vi "unit.vi"(8 "Error In":errorcluster, 9 "Signal Amp":dbl format="%#_7f", 11 "Unit":string) -> (0 "Error Out":errorcluster)   [LabVIEW 2021, in "Signal.lvlib"]
doc: "This subVI is used to check the unit value range and to enter the values to the signal_values_FGV."
uses:
  Signal.lvlib
  Tipski Definicii/rel_error.ctl
  Tipski Definicii/Unit.ctl
  Tipski Definicii/Signal Values.ctl
panel:
  # "Input"
  # "Output"
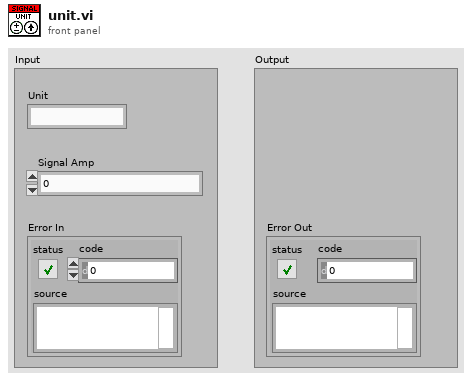
[diagram p1: front panel]
types:
  T1 = typedef "Unit.ctl" = enum16{"Init", "Add", "Read"}
  T2 = typedef "rel_error.ctl" = enum16{"Init", "Add String", "Error", "Get Error and Strings", "Reset"}
  T3 = typedef "Signal Values.ctl" = enum16{"Init", "Add V/A string", "Add Hz string", "Get Strings and Values", "Reset", "Add Offset", "Add Waveform", "Add Phase"}
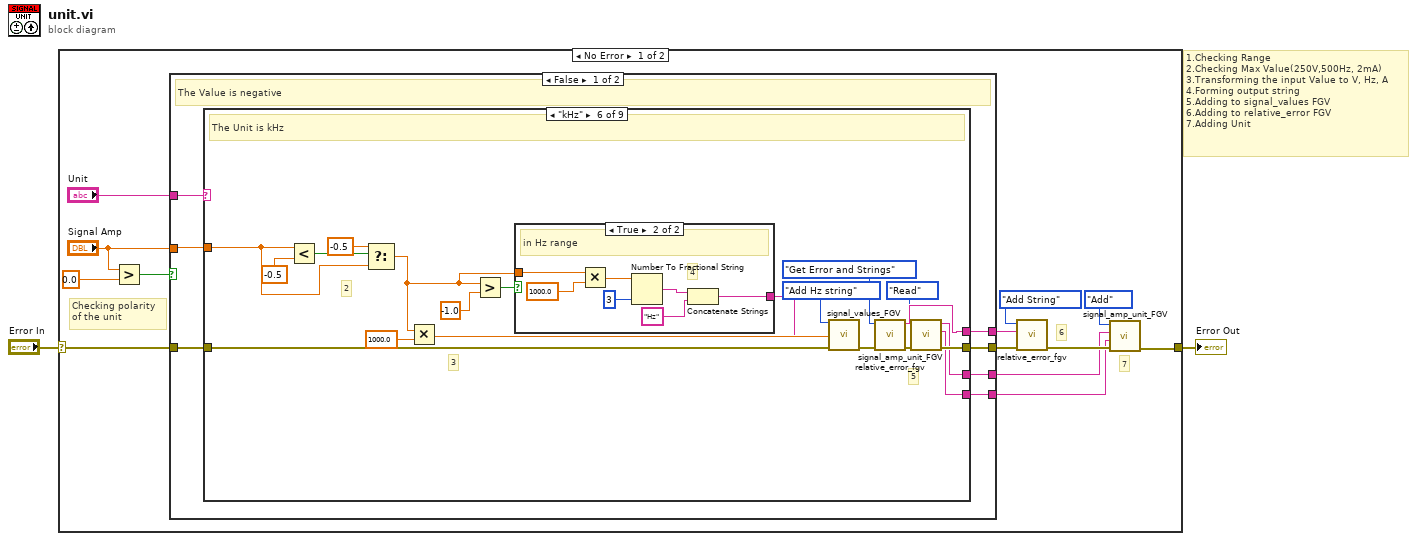
[diagram p0: block diagram]
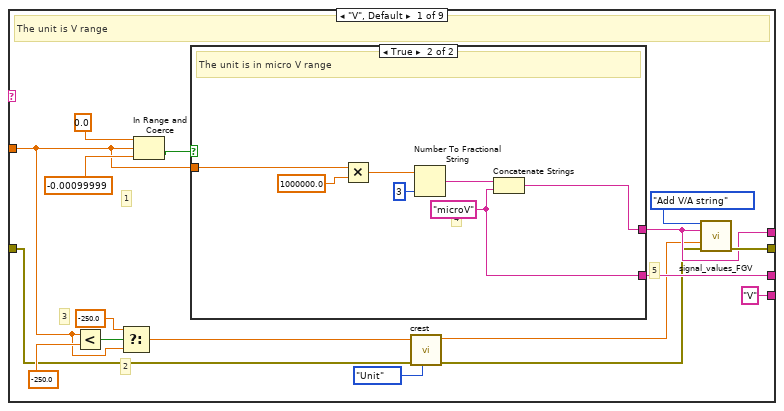
[diagram p2: hidden frame]
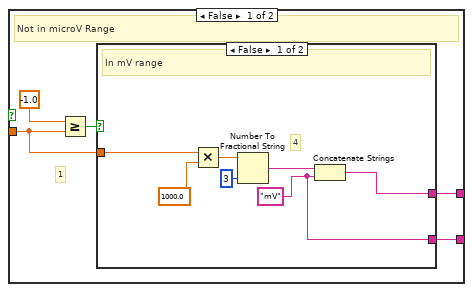
[diagram p3: hidden frame]
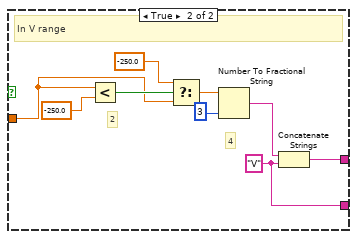
[diagram p4: hidden frame]
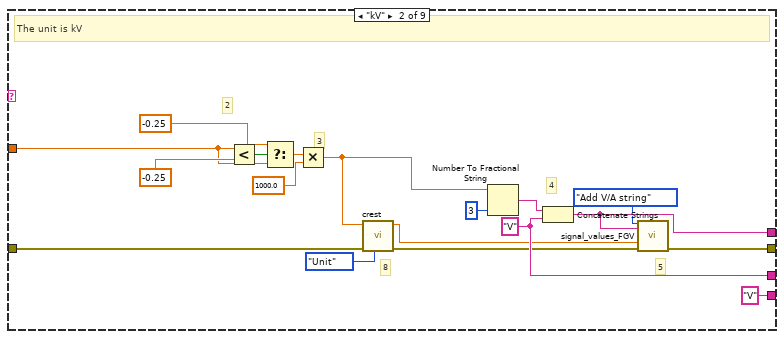
[diagram p5: hidden frame]
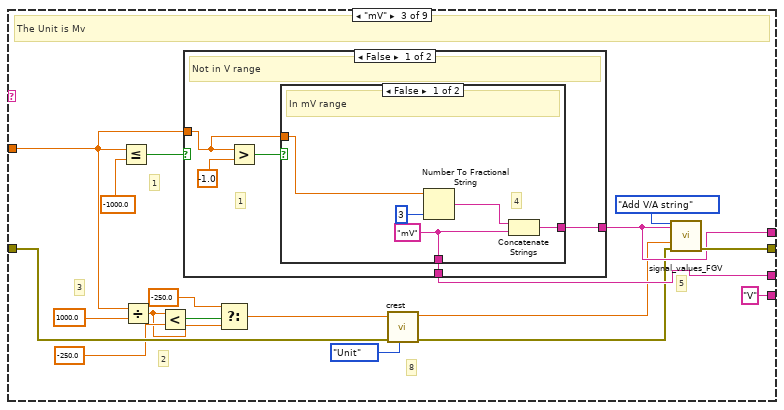
[diagram p6: hidden frame]
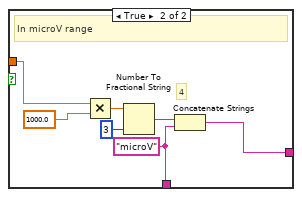
[diagram p7: hidden frame]
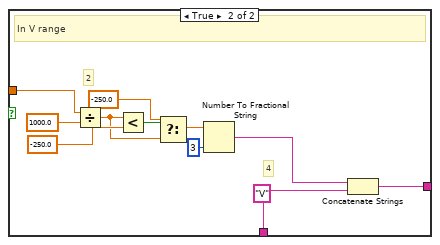
[diagram p8: hidden frame]
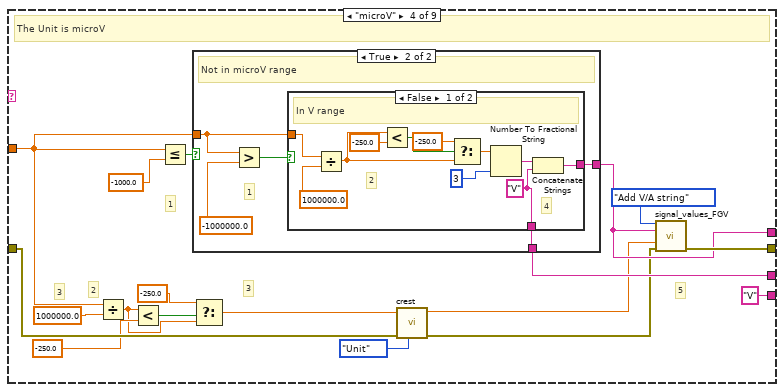
[diagram p9: hidden frame]
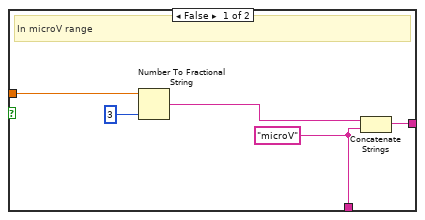
[diagram p10: hidden frame]
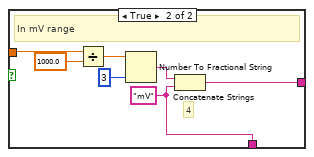
[diagram p11: hidden frame]
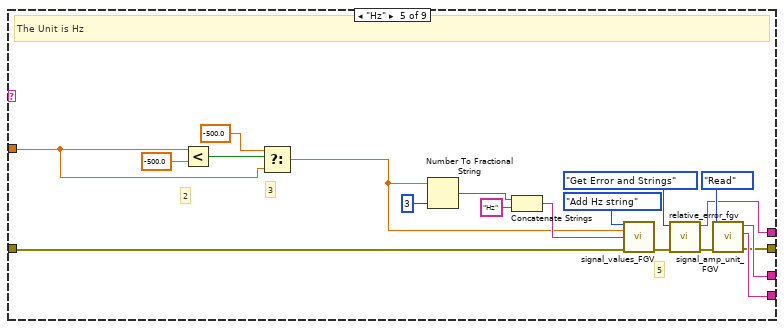
[diagram p12: hidden frame]
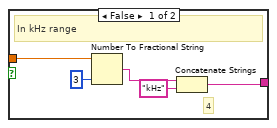
[diagram p13: hidden frame]
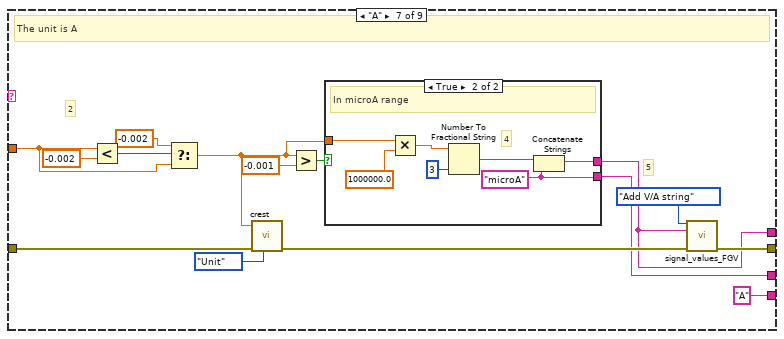
[diagram p14: hidden frame]
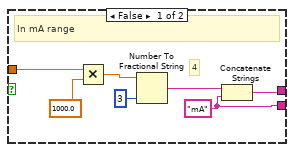
[diagram p15: hidden frame]
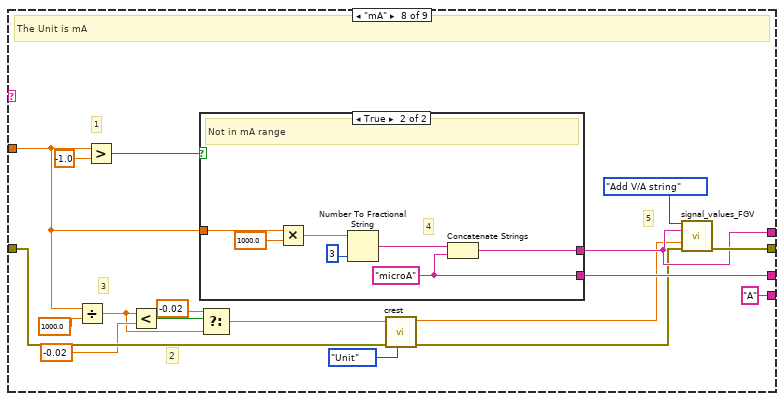
[diagram p16: hidden frame]
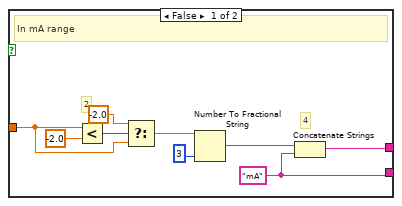
[diagram p17: hidden frame]
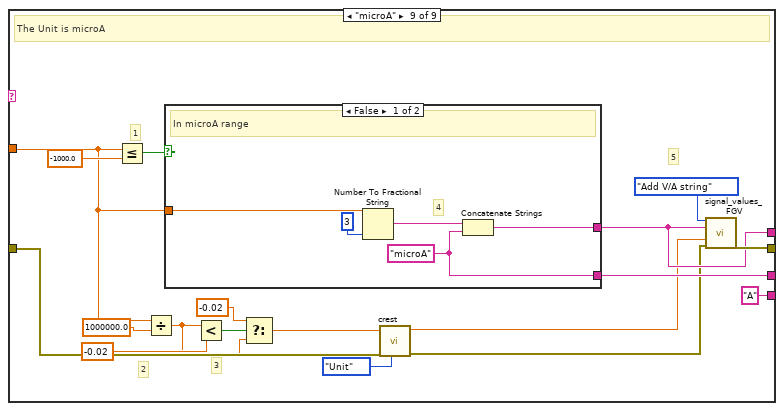
[diagram p18: hidden frame]
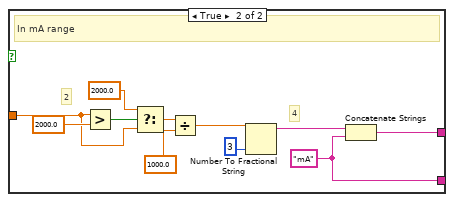
[diagram p19: hidden frame]
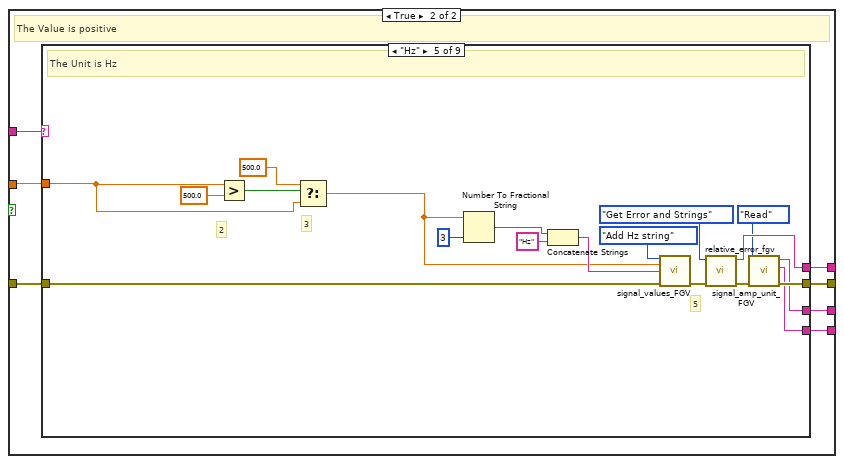
[diagram p20: hidden frame]
diagram:
  # "1.Checking Range\n2.Checking Max Value(250V,500Hz, 2mA)\n3.Transforming the input Value to V, Hz, A\n4.Forming output string\n5.Adding to signal_values FGV\n6.Adding to relative_error FGV\n7.Adding Unit"
  n1 = case shown="No Error" "Error In" {
    selector: "Error In" -> [w14 w636]
    tunnel: [w4 w636] -> w1
    frame No Error {
      # "7"
      # "6"
      # "Checking polarity\nof the unit"
      n2 = Greater?(x="Signal Amp", y=0.0) -> (0:w12:bool)
      n3 = case shown="False" w12 {
        tunnel: "Unit" -> [w20 w332]
        tunnel: w14 -> [w22 w330]
        tunnel: "Signal Amp" -> [w21 w331]
        tunnel: [w18 w329] -> w10
        tunnel: [w17 w328] -> w9
        tunnel: [w19 w327] -> w5
        tunnel: [w16 w326] -> w3
        frame False {
          # "The Value is negative"
          n4 = case shown="\"kHz\"" w20 {
            tunnel: [w36 w85 w99 w146 w179 w201 w231 w272 w306] -> w18
            tunnel: w21 -> [w29 w81 w94 w140 w183 w206 w234 w269 w302]
            tunnel: w22 -> [w28 w73 w103 w149 w182 w207 w235 w275 w309]
            tunnel: [w35 w76 w93 w139 w178 w199 w230 w268 w301] -> w17
            tunnel: [w34 w75 w92 w138 w180 w200 w232 w267 w304] -> w19
            tunnel: ["V" ("Base") "V" ("Base") "V" ("Base") "V" ("Base") w181 w197 "A" ("Base") "A" ("Base") "A" ("Base")] -> w16
            frame "V", Default {
              # "3"
              # "2"
              # "5"
              # "1"
              # "The unit is V range"
              n5 = Less?(x=w29, y=-250.0) -> (x < y?=w31:bool)
              n6 = Select(t=-250.0, s=w31, f=w29) -> (s? t:f=w27:dbl)
              n7 = In Range and Coerce(upper limit=0.0, x=w29, lower limit=-0.00099999) -> (In Range?=w39:bool)  [unwired: 1 out]
              n8 = case shown="True" w39 {
                tunnel: w29 -> [w42 w67]
                tunnel: [w41 w63] -> w35
                tunnel: [w40 w62] -> w34
                frame False {
                  # "1"
                  # "Not in microV Range"
                  n9 = Greater Or Equal?(x=-1.0, y=w42) -> (x >= y?=w43:bool)
                  n10 = case shown="False" w43 {
                    tunnel: w42 -> [w51 w56]
                    tunnel: [w47 w54] -> w41
                    tunnel: [w46 w53] -> w40
                    frame False {
                      w46 = "mV" ("string")
                      # "4"
                      # "In mV range"
                      n11 = Multiply(x=w51, y=1000.0) -> (x*y=w45:dbl)
                      n12 = Number To Fractional String(number=w45, precision (6)=i16 3) -> (F-format string=w48:string)  [unwired: 2 in]
                      n13 = Concatenate Strings(w48, w46) -> (w47:string)
                    }
                    frame True {
                      w53 = "V" ("string")
                      # "2"
                      # "4"
                      # "In V range"
                      n14 = Less?(x=w56, y=-250.0) -> (x < y?=w59:bool)
                      n15 = Select(t=-250.0, s=w59, f=w56) -> (s? t:f=w52:dbl)
                      n16 = Number To Fractional String(number=w52, precision (6)=i16 3) -> (F-format string=w55:string)  [unwired: 2 in]
                      n17 = Concatenate Strings(w55, w53) -> (w54:string)
                    }
                  }
                }
                frame True {
                  w62 = "microV" ("string")
                  # "4"
                  # "The unit is in micro V range"
                  n18 = Multiply(x=w67, y=1000000.0) -> (x*y=w61:dbl)
                  n19 = Number To Fractional String(number=w61, precision (6)=i16 3) -> (F-format string=w64:string)  [unwired: 2 in]
                  n20 = Concatenate Strings(w64, w62) -> (w63:string)
                }
              }
              n21 = call "crest.vi"("Set / Unit?"=enum16{"Unit", "SetUp"}."Unit", "Error In"=w28, "RMS"=w27) -> ("Error Out"=w25:errorcluster, "Max"=w26:dbl)  [unwired: 7 in]
              n22 = call "signal_values_FGV.vi"("Action"=Signal_Values."Add V/A string", "Amp String"=w35, "Amp Value"=w26, "Error In"=w25) -> ("Error Out"=w36:errorcluster)  [unwired: 10 in, 1 out]
            }
            frame "kV" {
              w75 = "V" ("string")
              # "8"
              # "2"
              # "5"
              # "4"
              # "3"
              # "The unit is kV"
              n23 = Less?(x=w81, y=-0.25) -> (x < y?=w83:bool)
              n24 = Select(t=-0.25, s=w83, f=w81) -> (s? t:f=w80:dbl)
              n25 = Multiply(x=w80, y=1000.0) -> (x*y=w72:dbl)
              n26 = call "crest.vi"("Set / Unit?"=enum16{"Unit", "SetUp"}."Unit", "Error In"=w73, "RMS"=w72) -> ("Error Out"=w71:errorcluster, "Max"=w70:dbl)  [unwired: 7 in]
              n27 = Number To Fractional String(number=w72, precision (6)=i16 3) -> (F-format string=w77:string)  [unwired: 2 in]
              n28 = Concatenate Strings(w77, w75) -> (w76:string)
              n29 = call "signal_values_FGV.vi"("Action"=Signal_Values."Add V/A string", "Amp String"=w76, "Amp Value"=w70, "Error In"=w71) -> ("Error Out"=w85:errorcluster)  [unwired: 10 in, 1 out]
            }
            frame "mV" {
              # "8"
              # "5"
              # "1"
              # "3"
              # "2"
              # "The Unit is Mv"
              n30 = Less Or Equal?(x=w94, y=-1000.0) -> (x <= y?=w101:bool)
              n31 = Divide(x=w94, y=1000.0) -> (x/y=w95:dbl)
              n32 = Less?(x=w95, y=-250.0) -> (x < y?=w97:bool)
              n33 = case shown="False" w101 {
                tunnel: w94 -> [w106 w124]
                tunnel: [w105 w122] -> w93
                tunnel: [w104 w121] -> w92
                frame False {
                  # "1"
                  # "Not in V range"
                  n34 = Greater?(x=w106, y=-1.0) -> (0:w107:bool)
                  n35 = case shown="False" w107 {
                    tunnel: w106 -> [w110 w120]
                    tunnel: [w112 w116] -> w105
                    tunnel: [w109 w114] -> w104
                    frame False {
                      w109 = "mV" ("string")
                      # "4"
                      # "In mV range"
                      n36 = Number To Fractional String(number=w110, precision (6)=i16 3) -> (F-format string=w111:string)  [unwired: 2 in]
                      n37 = Concatenate Strings(w111, w109) -> (w112:string)
                    }
                    frame True {
                      w114 = "microV" ("string")
                      # "4"
                      # "In microV range"
                      n38 = Multiply(x=w120, y=1000.0) -> (x*y=w115:dbl)
                      n39 = Number To Fractional String(number=w115, precision (6)=i16 3) -> (F-format string=w117:string)  [unwired: 2 in]
                      n40 = Concatenate Strings(w117, w114) -> (w116:string)
                    }
                  }
                }
                frame True {
                  w121 = "V" ("string")
                  # "2"
                  # "4"
                  # "In V range"
                  n41 = Divide(x=w124, y=1000.0) -> (x/y=w125:dbl)
                  n42 = Less?(x=w125, y=-250.0) -> (x < y?=w127:bool)
                  n43 = Select(t=-250.0, s=w127, f=w125) -> (s? t:f=w123:dbl)
                  n44 = Number To Fractional String(number=w123, precision (6)=i16 3) -> (F-format string=w129:string)  [unwired: 2 in]
                  n45 = Concatenate Strings(w129, w121) -> (w122:string)
                }
              }
              n46 = Select(t=-250.0, s=w97, f=w95) -> (s? t:f=w90:dbl)
              n47 = call "crest.vi"("Set / Unit?"=enum16{"Unit", "SetUp"}."Unit", "Error In"=w103, "RMS"=w90) -> ("Error Out"=w88:errorcluster, "Max"=w89:dbl)  [unwired: 7 in]
              n48 = call "signal_values_FGV.vi"("Action"=Signal_Values."Add V/A string", "Amp String"=w93, "Amp Value"=w89, "Error In"=w88) -> ("Error Out"=w99:errorcluster)  [unwired: 10 in, 1 out]
            }
            frame "microV" {
              # "3"
              # "5"
              # "1"
              # "3"
              # "2"
              # "The Unit is microV"
              n49 = Divide(x=w140, y=1000000.0) -> (x/y=w141:dbl)
              n50 = Less?(x=w141, y=-250.0) -> (x < y?=w143:bool)
              n51 = Less Or Equal?(x=w140, y=-1000.0) -> (x <= y?=w147:bool)
              n52 = case shown="True" w147 {
                tunnel: [w152 w157] -> w139
                tunnel: w140 -> [w151 w156]
                tunnel: [w150 w155] -> w138
                frame False {
                  w150 = "microV" ("string")
                  # "In microV range"
                  n53 = Number To Fractional String(number=w151, precision (6)=i16 3) -> (F-format string=w154:string)  [unwired: 2 in]
                  n54 = Concatenate Strings(w154, w150) -> (w152:string)
                }
                frame True {
                  # "1"
                  # "Not in microV range"
                  n55 = Greater?(x=w156, y=-1000000.0) -> (0:w158:bool)
                  n56 = case shown="False" w158 {
                    tunnel: [w164 w176] -> w157
                    tunnel: w156 -> [w162 w173]
                    tunnel: [w160 w171] -> w155
                    frame False {
                      w160 = "V"
                      # "2"
                      # "4"
                      # "In V range"
                      n57 = Divide(x=w162, y=1000000.0) -> (x/y=w166:dbl)
                      n58 = Less?(x=w166, y=-250.0) -> (x < y?=w168:bool)
                      n59 = Select(t=-250.0, s=w168, f=w166) -> (s? t:f=w161:dbl)
                      n60 = Number To Fractional String(number=w161, precision (6)=i16 3) -> (F-format string=w165:string)  [unwired: 2 in]
                      n61 = Concatenate Strings(w165, w160) -> (w164:string)
                    }
                    frame True {
                      w171 = "mV"
                      # "4"
                      # "In mV range"
                      n62 = Divide(x=w173, y=1000.0) -> (x/y=w172:dbl)
                      n63 = Number To Fractional String(number=w172, precision (6)=i16 3) -> (F-format string=w175:string)  [unwired: 2 in]
                      n64 = Concatenate Strings(w175, w171) -> (w176:string)
                    }
                  }
                }
              }
              n65 = Select(t=-250.0, s=w143, f=w141) -> (s? t:f=w136:dbl)
              n66 = call "crest.vi"("Set / Unit?"=enum16{"Unit", "SetUp"}."Unit", "Error In"=w149, "RMS"=w136) -> ("Error Out"=w134:errorcluster, "Max"=w135:dbl)  [unwired: 7 in]
              n67 = call "signal_values_FGV.vi"("Action"=Signal_Values."Add V/A string", "Amp String"=w139, "Amp Value"=w135, "Error In"=w134) -> ("Error Out"=w146:errorcluster)  [unwired: 10 in, 1 out]
            }
            frame "Hz" {
              # "5"
              # "3"
              # "2"
              # "The Unit is Hz"
              n68 = Less?(x=w183, y=-500.0) -> (x < y?=w195:bool)
              n69 = Select(t=-500.0 ("y"), s=w195, f=w183) -> (s? t:f=w184:dbl)
              n70 = Number To Fractional String(number=w184, precision (6)=i16 3) -> (F-format string=w186:string)  [unwired: 2 in]
              n71 = Concatenate Strings(w186, "Hz" ("string")) -> (w185:string)
              n72 = call "signal_values_FGV.vi"("Action"=Signal_Values."Add Hz string", "Hz Value"=w184, "Hz String"=w185, "Error In"=w182) -> ("Error Out"=w193:errorcluster)  [unwired: 10 in, 1 out]
              n73 = call "relative_error_fgv.vi"("Error In"=w193, "Action"=rel_error."Get Error and Strings") -> ("Error Out"=w190:errorcluster, "Starting String"=w178:string)  [unwired: 5 in, 3 out]
              n74 = call "signal_amp_unit_FGV.vi"("Error In"=w190, "Action"=Unit."Read") -> ("Error Out"=w179:errorcluster, "Base"=w181:string, "Unit (Not F)"=w180:string)  [unwired: 7 in]
            }
            frame "kHz" {
              # "5"
              # "3"
              # "2"
              # "The Unit is kHz"
              n75 = Less?(x=w206, y=-0.5) -> (x < y?=w215:bool)
              n76 = Select(t=-0.5, s=w215, f=w206) -> (s? t:f=w209:dbl)
              n77 = Multiply(x=w209, y=1000.0) -> (x*y=w212:dbl)
              n78 = Greater?(x=w209, y=-1.0) -> (0:w210:bool)
              n79 = case shown="True" w210 {
                tunnel: w209 -> [w221 w227]
                tunnel: [w217 w223] -> w208
                frame False {
                  # "4"
                  # "In kHz range"
                  n80 = Number To Fractional String(number=w221, precision (6)=i16 3) -> (F-format string=w219:string)  [unwired: 2 in]
                  n81 = Concatenate Strings(w219, "kHz" ("string")) -> (w217:string)
                }
                frame True {
                  # "4"
                  # "in Hz range"
                  n82 = Multiply(x=w227, y=1000.0) -> (x*y=w225:dbl)
                  n83 = Number To Fractional String(number=w225, precision (6)=i16 3) -> (F-format string=w228:string)  [unwired: 2 in]
                  n84 = Concatenate Strings(w228, "Hz" ("string")) -> (w223:string)
                }
              }
              n85 = call "signal_values_FGV.vi"("Action"=Signal_Values."Add Hz string", "Hz Value"=w212, "Hz String"=w208, "Error In"=w207) -> ("Error Out"=w205:errorcluster)  [unwired: 10 in, 1 out]
              n86 = call "relative_error_fgv.vi"("Error In"=w205, "Action"=rel_error."Get Error and Strings") -> ("Error Out"=w202:errorcluster, "Starting String"=w199:string)  [unwired: 5 in, 3 out]
              n87 = call "signal_amp_unit_FGV.vi"("Error In"=w202, "Action"=Unit."Read") -> ("Error Out"=w201:errorcluster, "Base"=w197:string, "Unit (Not F)"=w200:string)  [unwired: 7 in]
            }
            frame "A" {
              # "5"
              # "2"
              # "The unit is A"
              n88 = Less?(x=w234, y=-0.002) -> (x < y?=w242:bool)
              n89 = Select(t=-0.002, s=w242, f=w234) -> (s? t:f=w236:dbl)
              n90 = call "crest.vi"("Set / Unit?"=enum16{"Unit", "SetUp"}."Unit", "Error In"=w235, "RMS"=w236) -> ("Error Out"=w239:errorcluster)  [unwired: 7 in, 1 out]
              n91 = Greater?(x=w236, y=-0.001) -> (0:w237:bool)
              n92 = case shown="True" w237 {
                tunnel: [w245 w255] -> w232
                tunnel: [w244 w254] -> w230
                tunnel: w236 -> [w246 w253]
                frame False {
                  w245 = "mA" ("string")
                  # "4"
                  # "In mA range"
                  n93 = Multiply(x=w246, y=1000.0) -> (x*y=w248:dbl)
                  n94 = Number To Fractional String(number=w248, precision (6)=i16 3) -> (F-format string=w249:string)  [unwired: 2 in]
                  n95 = Concatenate Strings(w249, w245) -> (w244:string)
                }
                frame True {
                  w255 = "microA" ("string")
                  # "4"
                  # "In microA range"
                  n96 = Multiply(x=w253, y=1000000.0) -> (x*y=w252:dbl)
                  n97 = Number To Fractional String(number=w252, precision (6)=i16 3) -> (F-format string=w256:string)  [unwired: 2 in]
                  n98 = Concatenate Strings(w256, w255) -> (w254:string)
                }
              }
              n99 = call "signal_values_FGV.vi"("Action"=Signal_Values."Add V/A string", "Amp String"=w230, "Error In"=w239) -> ("Error Out"=w231:errorcluster)  [unwired: 11 in, 1 out]
            }
            frame "mA" {
              # "3"
              # "2"
              # "5"
              # "1"
              # "The Unit is mA"
              n100 = Divide(x=w269, y=1000.0) -> (x/y=w263:dbl)
              n101 = Greater?(x=w269, y=-1.0) -> (0:w273:bool)
              n102 = Less?(x=w263, y=-0.02) -> (x < y?=w265:bool)
              n103 = case shown="True" w273 {
                tunnel: w269 -> [w282 w291]
                tunnel: [w277 w287] -> w268
                tunnel: [w276 w286] -> w267
                frame False {
                  w276 = "mA" ("string")
                  # "4"
                  # "2"
                  # "In mA range"
                  n104 = Less?(x=w282, y=-2.0) -> (x < y?=w283:bool)
                  n105 = Select(t=-2.0, s=w283, f=w282) -> (s? t:f=w278:dbl)
                  n106 = Number To Fractional String(number=w278, precision (6)=i16 3) -> (F-format string=w279:string)  [unwired: 2 in]
                  n107 = Concatenate Strings(w279, w276) -> (w277:string)
                }
                frame True {
                  w286 = "microA" ("string")
                  # "4"
                  # "Not in mA range"
                  n108 = Multiply(x=w291, y=1000.0) -> (x*y=w288:dbl)
                  n109 = Number To Fractional String(number=w288, precision (6)=i16 3) -> (F-format string=w285:string)  [unwired: 2 in]
                  n110 = Concatenate Strings(w285, w286) -> (w287:string)
                }
              }
              n111 = Select(t=-0.02, s=w265, f=w263) -> (s? t:f=w261:dbl)
              n112 = call "crest.vi"("Set / Unit?"=enum16{"Unit", "SetUp"}."Unit", "Error In"=w275, "RMS"=w261) -> ("Error Out"=w262:errorcluster, "Max"=w260:dbl)  [unwired: 7 in]
              n113 = call "signal_values_FGV.vi"("Action"=Signal_Values."Add V/A string", "Amp String"=w268, "Amp Value"=w260, "Error In"=w262) -> ("Error Out"=w272:errorcluster)  [unwired: 10 in, 1 out]
            }
            frame "microA" {
              # "2"
              # "5"
              # "3"
              # "1"
              # "The Unit is microA"
              n114 = Less Or Equal?(x=w302, y=-1000.0) -> (x <= y?=w307:bool)
              n115 = Divide(x=w302, y=1000000.0) -> (x/y=w297:dbl)
              n116 = case shown="False" w307 {
                tunnel: w302 -> [w310 w322]
                tunnel: [w312 w316] -> w301
                tunnel: [w311 w315] -> w304
                frame False {
                  w311 = "microA" ("string")
                  # "4"
                  # "In microA range"
                  n117 = Number To Fractional String(number=w310, precision (6)=i16 3) -> (F-format string=w313:string)  [unwired: 2 in]
                  n118 = Concatenate Strings(w313, w311) -> (w312:string)
                }
                frame True {
                  w315 = "mA" ("string")
                  # "2"
                  # "4"
                  # "In mA range"
                  n119 = Greater?(x=w322, y=2000.0) -> (0:w324:bool)
                  n120 = Select(t=2000.0, s=w324, f=w322) -> (s? t:f=w321:dbl)
                  n121 = Divide(x=w321, y=1000.0) -> (x/y=w317:dbl)
                  n122 = Number To Fractional String(number=w317, precision (6)=i16 3) -> (F-format string=w318:string)  [unwired: 2 in]
                  n123 = Concatenate Strings(w318, w315) -> (w316:string)
                }
              }
              n124 = Less?(x=w297, y=-0.02) -> (x < y?=w299:bool)
              n125 = Select(t=-0.02, s=w299, f=w297) -> (s? t:f=w296:dbl)
              n126 = call "crest.vi"("Set / Unit?"=enum16{"Unit", "SetUp"}."Unit", "Error In"=w309, "RMS"=w296) -> ("Error Out"=w294:errorcluster, "Max"=w295:dbl)  [unwired: 7 in]
              n127 = call "signal_values_FGV.vi"("Action"=Signal_Values."Add V/A string", "Amp String"=w301, "Amp Value"=w295, "Error In"=w294) -> ("Error Out"=w306:errorcluster)  [unwired: 10 in, 1 out]
            }
          }
        }
        frame True {
          # "The Value is positive"
          n128 = case shown="\"Hz\"" w332 {
            tunnel: [w346 w395 w409 w456 w497 w511 w549 w582 w616] -> w329
            tunnel: w331 -> [w339 w391 w404 w450 w503 w516 w550 w579 w612]
            tunnel: w330 -> [w338 w383 w413 w459 w502 w517 w545 w585 w619]
            tunnel: [w345 w386 w403 w449 w496 w509 w546 w578 w611] -> w328
            tunnel: [w344 w385 w402 w448 w494 w510 w547 w577 w614] -> w327
            tunnel: ["V" ("string") "V" ("string") "V" ("string") "V" ("string") w493 w507 "A" ("Base") "A" ("Base") "A" ("Base")] -> w326
            frame "V", Default {
              # "3"
              # "2"
              # "5"
              # "1"
              # "The unit is V range"
              n129 = Greater?(x=w339, y=250.0) -> (0:w341:bool)
              n130 = Select(t=250.0, s=w341, f=w339) -> (s? t:f=w337:dbl)
              n131 = In Range and Coerce(upper limit=1.0, x=w339, lower limit=0.001) -> (In Range?=w349:bool)  [unwired: 1 out]
              n132 = case shown="False" w349 {
                tunnel: w339 -> [w352 w377]
                tunnel: [w351 w373] -> w345
                tunnel: [w350 w372] -> w344
                frame False {
                  # "1"
                  # "Not in mV range"
                  n133 = Less?(x=0.001, y=w352) -> (x < y?=w353:bool)
                  n134 = case shown="False" w353 {
                    tunnel: w352 -> [w361 w366]
                    tunnel: [w357 w364] -> w351
                    tunnel: [w356 w363] -> w350
                    frame False {
                      w356 = "microV" ("string")
                      # "4"
                      # "In microV range"
                      n135 = Multiply(x=w361, y=1000000.0) -> (x*y=w355:dbl)
                      n136 = Number To Fractional String(number=w355, precision (6)=i16 3) -> (F-format string=w358:string)  [unwired: 2 in]
                      n137 = Concatenate Strings(w358, w356) -> (w357:string)
                    }
                    frame True {
                      w363 = "V" ("string")
                      # "2"
                      # "4"
                      # "In V range"
                      n138 = Greater?(x=w366, y=250.0) -> (0:w369:bool)
                      n139 = Select(t=250.0, s=w369, f=w366) -> (s? t:f=w362:dbl)
                      n140 = Number To Fractional String(number=w362, precision (6)=i16 3) -> (F-format string=w365:string)  [unwired: 2 in]
                      n141 = Concatenate Strings(w365, w363) -> (w364:string)
                    }
                  }
                }
                frame True {
                  w372 = "mV" ("string")
                  # "4"
                  # "The unit is in mV range"
                  n142 = Multiply(x=w377, y=1000.0) -> (x*y=w371:dbl)
                  n143 = Number To Fractional String(number=w371, precision (6)=i16 3) -> (F-format string=w374:string)  [unwired: 2 in]
                  n144 = Concatenate Strings(w374, w372) -> (w373:string)
                }
              }
              n145 = call "crest.vi"("Set / Unit?"=enum16{"Unit", "SetUp"}."Unit", "Error In"=w338, "RMS"=w337) -> ("Error Out"=w335:errorcluster, "Max"=w336:dbl)  [unwired: 7 in]
              n146 = call "signal_values_FGV.vi"("Action"=Signal_Values."Add V/A string", "Amp String"=w345, "Amp Value"=w336, "Error In"=w335) -> ("Error Out"=w346:errorcluster)  [unwired: 10 in, 1 out]
            }
            frame "kV" {
              w385 = "V" ("string")
              # "8"
              # "2"
              # "5"
              # "4"
              # "3"
              # "Kv Unit"
              n147 = Greater?(x=w391, y=0.25) -> (0:w393:bool)
              n148 = Select(t=0.25, s=w393, f=w391) -> (s? t:f=w390:dbl)
              n149 = Multiply(x=w390, y=1000.0) -> (x*y=w382:dbl)
              n150 = call "crest.vi"("Set / Unit?"=enum16{"Unit", "SetUp"}."Unit", "Error In"=w383, "RMS"=w382) -> ("Error Out"=w381:errorcluster, "Max"=w380:dbl)  [unwired: 7 in]
              n151 = Number To Fractional String(number=w382, precision (6)=i16 3) -> (F-format string=w387:string)  [unwired: 2 in]
              n152 = Concatenate Strings(w387, w385) -> (w386:string)
              n153 = call "signal_values_FGV.vi"("Action"=Signal_Values."Add V/A string", "Amp String"=w386, "Amp Value"=w380, "Error In"=w381) -> ("Error Out"=w395:errorcluster)  [unwired: 10 in, 1 out]
            }
            frame "mV" {
              # "8"
              # "5"
              # "1"
              # "3"
              # "2"
              # "The Unit is Mv"
              n154 = Greater Or Equal?(x=w404, y=1000.0) -> (x >= y?=w411:bool)
              n155 = Divide(x=w404, y=1000.0) -> (x/y=w405:dbl)
              n156 = Greater?(x=w405, y=250.0) -> (0:w407:bool)
              n157 = case shown="False" w411 {
                tunnel: w404 -> [w416 w434]
                tunnel: [w415 w432] -> w403
                tunnel: [w414 w431] -> w402
                frame False {
                  # "1"
                  # "Not in V range"
                  n158 = Less?(x=w416, y=1.0) -> (x < y?=w417:bool)
                  n159 = case shown="True" w417 {
                    tunnel: w416 -> [w420 w430]
                    tunnel: [w422 w426] -> w415
                    tunnel: [w419 w424] -> w414
                    frame False {
                      w419 = "mV" ("string")
                      # "4"
                      # "In mV range"
                      n160 = Number To Fractional String(number=w420, precision (6)=i16 3) -> (F-format string=w421:string)  [unwired: 2 in]
                      n161 = Concatenate Strings(w421, w419) -> (w422:string)
                    }
                    frame True {
                      w424 = "microV" ("string")
                      # "4"
                      # "In microV range"
                      n162 = Multiply(x=w430, y=1000.0) -> (x*y=w425:dbl)
                      n163 = Number To Fractional String(number=w425, precision (6)=i16 3) -> (F-format string=w427:string)  [unwired: 2 in]
                      n164 = Concatenate Strings(w427, w424) -> (w426:string)
                    }
                  }
                }
                frame True {
                  w431 = "V" ("string")
                  # "2"
                  # "4"
                  # "In V range"
                  n165 = Divide(x=w434, y=1000.0) -> (x/y=w435:dbl)
                  n166 = Greater?(x=w435, y=250.0) -> (0:w437:bool)
                  n167 = Select(t=250.0, s=w437, f=w435) -> (s? t:f=w433:dbl)
                  n168 = Number To Fractional String(number=w433, precision (6)=i16 3) -> (F-format string=w439:string)  [unwired: 2 in]
                  n169 = Concatenate Strings(w439, w431) -> (w432:string)
                }
              }
              n170 = Select(t=250.0, s=w407, f=w405) -> (s? t:f=w400:dbl)
              n171 = call "crest.vi"("Set / Unit?"=enum16{"Unit", "SetUp"}."Unit", "Error In"=w413, "RMS"=w400) -> ("Error Out"=w398:errorcluster, "Max"=w399:dbl)  [unwired: 7 in]
              n172 = call "signal_values_FGV.vi"("Action"=Signal_Values."Add V/A string", "Amp String"=w403, "Amp Value"=w399, "Error In"=w398) -> ("Error Out"=w409:errorcluster)  [unwired: 10 in, 1 out]
            }
            frame "microV" {
              # "3"
              # "5"
              # "1"
              # "3"
              # "2"
              # "The Unit is microV"
              n173 = Divide(x=w450, y=1000000.0) -> (x/y=w451:dbl)
              n174 = Greater?(x=w451, y=250.0) -> (0:w453:bool)
              n175 = Greater Or Equal?(x=w450, y=1000.0) -> (x >= y?=w457:bool)
              n176 = case shown="True" w457 {
                tunnel: [w462 w467] -> w449
                tunnel: w450 -> [w461 w466]
                tunnel: [w460 w465] -> w448
                frame False {
                  w460 = "microV" ("string")
                  # "In microV range"
                  n177 = Number To Fractional String(number=w461, precision (6)=i16 3) -> (F-format string=w464:string)  [unwired: 2 in]
                  n178 = Concatenate Strings(w464, w460) -> (w462:string)
                }
                frame True {
                  # "1"
                  # "Not in microV range"
                  n179 = Less?(x=w466, y=1000000.0) -> (x < y?=w468:bool)
                  n180 = case shown="True" w468 {
                    tunnel: [w474 w486] -> w467
                    tunnel: w466 -> [w472 w483]
                    tunnel: [w470 w481] -> w465
                    frame False {
                      w470 = "V"
                      # "2"
                      # "4"
                      # "In V range"
                      n181 = Divide(x=w472, y=1000000.0) -> (x/y=w476:dbl)
                      n182 = Greater?(x=w476, y=250.0) -> (0:w478:bool)
                      n183 = Select(t=250.0, s=w478, f=w476) -> (s? t:f=w471:dbl)
                      n184 = Number To Fractional String(number=w471, precision (6)=i16 3) -> (F-format string=w475:string)  [unwired: 2 in]
                      n185 = Concatenate Strings(w475, w470) -> (w474:string)
                    }
                    frame True {
                      w481 = "mV"
                      # "4"
                      # "In mV range"
                      n186 = Divide(x=w483, y=1000.0) -> (x/y=w482:dbl)
                      n187 = Number To Fractional String(number=w482, precision (6)=i16 3) -> (F-format string=w485:string)  [unwired: 2 in]
                      n188 = Concatenate Strings(w485, w481) -> (w486:string)
                    }
                  }
                }
              }
              n189 = Select(t=250.0, s=w453, f=w451) -> (s? t:f=w446:dbl)
              n190 = call "crest.vi"("Set / Unit?"=enum16{"Unit", "SetUp"}."Unit", "Error In"=w459, "RMS"=w446) -> ("Error Out"=w444:errorcluster, "Max"=w445:dbl)  [unwired: 7 in]
              n191 = call "signal_values_FGV.vi"("Action"=Signal_Values."Add V/A string", "Amp String"=w449, "Amp Value"=w445, "Error In"=w444) -> ("Error Out"=w456:errorcluster)  [unwired: 10 in, 1 out]
            }
            frame "Hz" {
              # "5"
              # "3"
              # "2"
              # "The Unit is Hz"
              n192 = Greater?(x=w503, y=500.0) -> (0:w505:bool)
              n193 = Select(t=500.0 ("y"), s=w505, f=w503) -> (s? t:f=w488:dbl)
              n194 = Number To Fractional String(number=w488, precision (6)=i16 3) -> (F-format string=w490:string)  [unwired: 2 in]
              n195 = Concatenate Strings(w490, "Hz" ("string")) -> (w489:string)
              n196 = call "signal_values_FGV.vi"("Action"=Signal_Values."Add Hz string", "Hz Value"=w488, "Hz String"=w489, "Error In"=w502) -> ("Error Out"=w501:errorcluster)  [unwired: 10 in, 1 out]
              n197 = call "relative_error_fgv.vi"("Error In"=w501, "Action"=rel_error."Get Error and Strings") -> ("Error Out"=w498:errorcluster, "Starting String"=w496:string)  [unwired: 5 in, 3 out]
              n198 = call "signal_amp_unit_FGV.vi"("Error In"=w498, "Action"=Unit."Read") -> ("Error Out"=w497:errorcluster, "Base"=w493:string, "Unit (Not F)"=w494:string)  [unwired: 7 in]
            }
            frame "kHz" {
              # "5"
              # "3"
              # "2"
              # "The Unit is kHz"
              n199 = Greater?(x=w516, y=0.5) -> (0:w525:bool)
              n200 = Select(t=0.5, s=w525, f=w516) -> (s? t:f=w519:dbl)
              n201 = Multiply(x=w519, y=1000.0) -> (x*y=w522:dbl)
              n202 = Less?(x=w519, y=1.0) -> (x < y?=w520:bool)
              n203 = case shown="True" w520 {
                tunnel: w519 -> [w531 w537]
                tunnel: [w527 w533] -> w518
                frame False {
                  # "4"
                  # "In kHz range"
                  n204 = Number To Fractional String(number=w531, precision (6)=i16 3) -> (F-format string=w529:string)  [unwired: 2 in]
                  n205 = Concatenate Strings(w529, "kHz" ("string")) -> (w527:string)
                }
                frame True {
                  # "4"
                  # "in Hz range"
                  n206 = Multiply(x=w537, y=1000.0) -> (x*y=w535:dbl)
                  n207 = Number To Fractional String(number=w535, precision (6)=i16 3) -> (F-format string=w538:string)  [unwired: 2 in]
                  n208 = Concatenate Strings(w538, "Hz" ("string")) -> (w533:string)
                }
              }
              n209 = call "signal_values_FGV.vi"("Action"=Signal_Values."Add Hz string", "Hz Value"=w522, "Hz String"=w518, "Error In"=w517) -> ("Error Out"=w515:errorcluster)  [unwired: 10 in, 1 out]
              n210 = call "relative_error_fgv.vi"("Error In"=w515, "Action"=rel_error."Get Error and Strings") -> ("Error Out"=w512:errorcluster, "Starting String"=w509:string)  [unwired: 5 in, 3 out]
              n211 = call "signal_amp_unit_FGV.vi"("Error In"=w512, "Action"=Unit."Read") -> ("Error Out"=w511:errorcluster, "Base"=w507:string, "Unit (Not F)"=w510:string)  [unwired: 7 in]
            }
            frame "A" {
              # "5"
              # "2"
              # "The unit is A"
              n212 = Greater?(x=w550, y=0.002) -> (0:w552:bool)
              n213 = Select(t=0.002, s=w552, f=w550) -> (s? t:f=w540:dbl)
              n214 = call "crest.vi"("Set / Unit?"=enum16{"Unit", "SetUp"}."Unit", "Error In"=w545, "RMS"=w540) -> ("Error Out"=w544:errorcluster)  [unwired: 7 in, 1 out]
              n215 = Less?(x=w540, y=0.001) -> (x < y?=w541:bool)
              n216 = case shown="True" w541 {
                tunnel: [w555 w565] -> w547
                tunnel: [w554 w564] -> w546
                tunnel: w540 -> [w556 w563]
                frame False {
                  w555 = "mA" ("string")
                  # "4"
                  # "In mA Range"
                  n217 = Multiply(x=w556, y=1000.0) -> (x*y=w558:dbl)
                  n218 = Number To Fractional String(number=w558, precision (6)=i16 3) -> (F-format string=w559:string)  [unwired: 2 in]
                  n219 = Concatenate Strings(w559, w555) -> (w554:string)
                }
                frame True {
                  w565 = "microA" ("string")
                  # "4"
                  # "In microA range"
                  n220 = Multiply(x=w563, y=1000000.0) -> (x*y=w562:dbl)
                  n221 = Number To Fractional String(number=w562, precision (6)=i16 3) -> (F-format string=w566:string)  [unwired: 2 in]
                  n222 = Concatenate Strings(w566, w565) -> (w564:string)
                }
              }
              n223 = call "signal_values_FGV.vi"("Action"=Signal_Values."Add V/A string", "Amp String"=w546, "Error In"=w544) -> ("Error Out"=w549:errorcluster)  [unwired: 11 in, 1 out]
            }
            frame "mA" {
              # "3"
              # "2"
              # "5"
              # "1"
              # "The Unit is mA"
              n224 = Divide(x=w579, y=1000.0) -> (x/y=w573:dbl)
              n225 = Less?(x=w579, y=1.0) -> (x < y?=w583:bool)
              n226 = Greater?(x=w573, y=0.02) -> (0:w575:bool)
              n227 = case shown="True" w583 {
                tunnel: w579 -> [w592 w601]
                tunnel: [w587 w597] -> w578
                tunnel: [w586 w596] -> w577
                frame False {
                  w586 = "mA" ("string")
                  # "4"
                  # "2"
                  # "In mA range"
                  n228 = Greater?(x=w592, y=2.0) -> (0:w593:bool)
                  n229 = Select(t=2.0, s=w593, f=w592) -> (s? t:f=w588:dbl)
                  n230 = Number To Fractional String(number=w588, precision (6)=i16 3) -> (F-format string=w589:string)  [unwired: 2 in]
                  n231 = Concatenate Strings(w589, w586) -> (w587:string)
                }
                frame True {
                  w596 = "microA" ("string")
                  # "4"
                  # "Not in mA range"
                  n232 = Multiply(x=w601, y=1000.0) -> (x*y=w598:dbl)
                  n233 = Number To Fractional String(number=w598, precision (6)=i16 3) -> (F-format string=w595:string)  [unwired: 2 in]
                  n234 = Concatenate Strings(w595, w596) -> (w597:string)
                }
              }
              n235 = Select(t=0.02, s=w575, f=w573) -> (s? t:f=w571:dbl)
              n236 = call "crest.vi"("Set / Unit?"=enum16{"Unit", "SetUp"}."Unit", "Error In"=w585, "RMS"=w571) -> ("Error Out"=w572:errorcluster, "Max"=w570:dbl)  [unwired: 7 in]
              n237 = call "signal_values_FGV.vi"("Action"=Signal_Values."Add V/A string", "Amp String"=w578, "Amp Value"=w570, "Error In"=w572) -> ("Error Out"=w582:errorcluster)  [unwired: 10 in, 1 out]
            }
            frame "microA" {
              # "2"
              # "5"
              # "3"
              # "1"
              # "The Unit is microA"
              n238 = Greater Or Equal?(x=w612, y=1000.0) -> (x >= y?=w617:bool)
              n239 = Divide(x=w612, y=1000000.0) -> (x/y=w607:dbl)
              n240 = case shown="True" w617 {
                tunnel: w612 -> [w620 w632]
                tunnel: [w622 w626] -> w611
                tunnel: [w621 w625] -> w614
                frame False {
                  w621 = "microA" ("string")
                  # "4"
                  # "In microA range"
                  n241 = Number To Fractional String(number=w620, precision (6)=i16 3) -> (F-format string=w623:string)  [unwired: 2 in]
                  n242 = Concatenate Strings(w623, w621) -> (w622:string)
                }
                frame True {
                  w625 = "mA" ("string")
                  # "2"
                  # "4"
                  # "In mA range"
                  n243 = Greater?(x=w632, y=2000.0) -> (0:w634:bool)
                  n244 = Select(t=2000.0, s=w634, f=w632) -> (s? t:f=w631:dbl)
                  n245 = Divide(x=w631, y=1000.0) -> (x/y=w627:dbl)
                  n246 = Number To Fractional String(number=w627, precision (6)=i16 3) -> (F-format string=w628:string)  [unwired: 2 in]
                  n247 = Concatenate Strings(w628, w625) -> (w626:string)
                }
              }
              n248 = Greater?(x=w607, y=0.02) -> (0:w609:bool)
              n249 = Select(t=0.02, s=w609, f=w607) -> (s? t:f=w606:dbl)
              n250 = call "crest.vi"("Set / Unit?"=enum16{"Unit", "SetUp"}."Unit", "Error In"=w619, "RMS"=w606) -> ("Error Out"=w604:errorcluster, "Max"=w605:dbl)  [unwired: 7 in]
              n251 = call "signal_values_FGV.vi"("Action"=Signal_Values."Add V/A string", "Amp String"=w611, "Amp Value"=w605, "Error In"=w604) -> ("Error Out"=w616:errorcluster)  [unwired: 10 in, 1 out]
            }
          }
        }
      }
      n252 = call "relative_error_fgv.vi"("Error In"=w10, "Amp String"=w9, "Action"=rel_error."Add String") -> ("Error Out"=w7:errorcluster)  [unwired: 4 in, 4 out]
      n253 = call "signal_amp_unit_FGV.vi"("Error In"=w7, "Base Unit"=w3, "Unit (Not F)"=w5, "Action"=Unit."Add") -> ("Error Out"=w4:errorcluster)  [unwired: 5 in, 2 out]
    }
    frame Error {
    }
  }
  "Error Out" <- w1
